vi "Get Controller State.vi"(8 "error in (no error)":errorcluster, 11 "ATM Controller in":refnum<class "ATM Controller.lvclass">) -> (0 "error out":errorcluster, 2 "ATM State":T1, 3 "ATM Controller out":refnum<class "ATM Controller.lvclass">)   [LabVIEW 2020, in "ATM Controller.lvclass"]
uses:
  ATM Controller.lvclass
  State.ctl
  ATM Controller.lvclass/ATM Controller.ctl
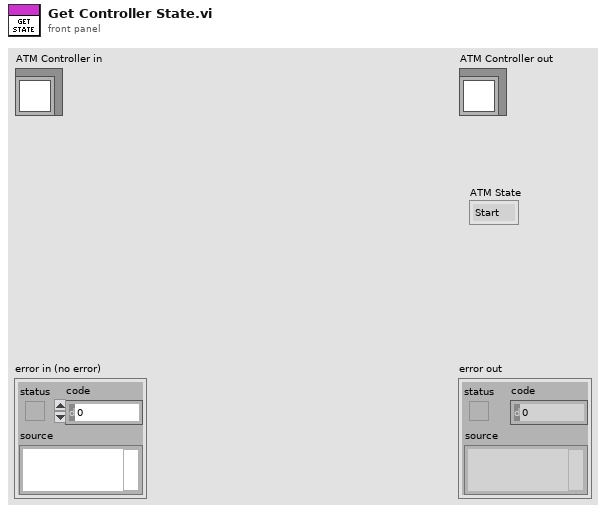
[diagram p1: front panel]
types:
  T1 = typedef "ATM Controller.lvclass/State.ctl" = enum16{"Start", "Insert Card", "Deposit", "Withdraw", "Fast Cash", "None", "Balance Inquiry", "Return Card"}
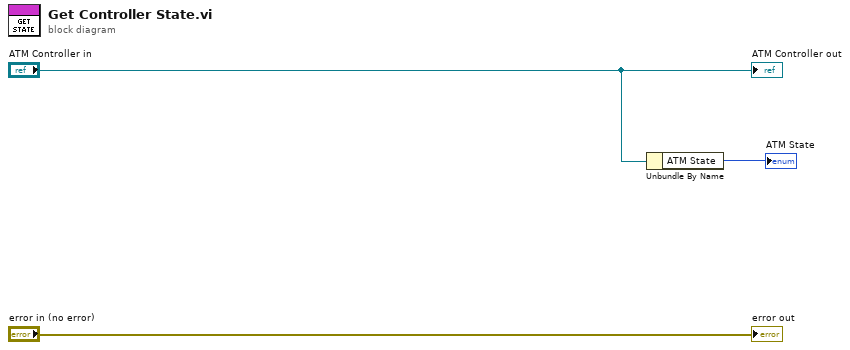
[diagram p0: block diagram]
diagram:
  n1 = Unbundle By Name("ATM Controller in") -> ("ATM State"=→"ATM State":T1)
  "error out" <- "error in (no error)"
  "ATM Controller out" <- "ATM Controller in"
